vi "Disconnect Core.vi"(8 "error in (no error)":errorcluster, 10 "Force (T)":bool=TRUE, 11 "BNT_SLTagConnection in":refnum<class "BNT_SLTagConnection.lvclass">) -> (0 "error out":errorcluster, 3 "BNT_SLTagConnection out":refnum<class "BNT_SLTagConnection.lvclass">)   [LabVIEW 2019, in "BNT_SLTagConnection.lvlib" / "BNT_SLTagConnection.lvclass"]
doc: "Close reference to a process variable."
uses:
  BNT_SLTagConnection.lvclass
  BNT_SLTagConnection.lvclass/BNT_SLTagConnection.ctl
  <vilib>/Skyline/Tag/Wrapper/Wrapper_class/NI Skyline Tag.lvclass/NI Skyline Tag.ctl
  <vilib>/Skyline/Tag/Wrapper/Wrapper_class/NI Skyline Tag.lvclass
  <vilib>/Skyline/Tag/Wrapper/Wrapper_class/Read Tag Path.vi
  <vilib>/Skyline/Tag/Wrapper/Wrapper_class/Close Tag (Single).vi
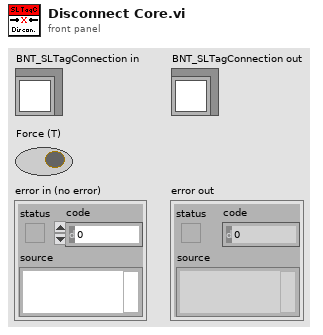
[diagram p1: front panel]
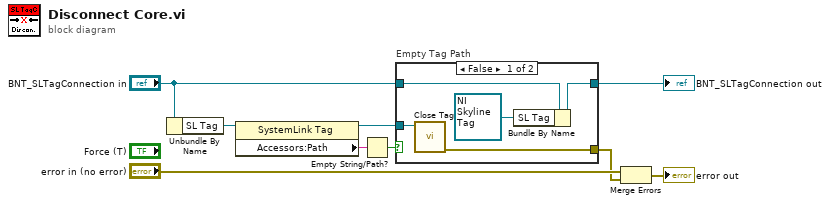
[diagram p0: block diagram]
diagram:
  n1 = Unbundle By Name("BNT_SLTagConnection in") -> ("SL Tag"=w3:refnum<class "NI Skyline Tag.lvclass">)
  n2 = property class="SystemLink Tag"(reference=w3) -> (reference out=w2:refnum<class "NI Skyline Tag.lvclass">, "Accessors:Path"=w1:string)  [unwired: 1 in, 1 out]
  n3 = Empty String/Path?(string/path=w1) -> (empty?=w7:bool)
  n4 = case "Empty Tag Path" shown="False" w7 {
    tunnel: w2 -> [w14 _]
    tunnel: [w13 _] -> w4
    tunnel: "BNT_SLTagConnection in" -> [w12 w15]
    tunnel: [w11 w15] -> w8
    frame False {
      n5 = call-poly <vilib>:"Close Tag.vi"("tag"=w14) -> ("error out"=w13:errorcluster)  [unwired: 10 in]
      n6 = Bundle By Name(cluster=w12, "SL Tag"=refnum<class "NI Skyline Tag.lvclass"> refnum ("Tag")) -> (w11:refnum<class "BNT_SLTagConnection.lvclass">)
    }
    frame True {
    }
  }
  "BNT_SLTagConnection out" <- w8
  n7 = Merge Errors("error in (no error)", w4) -> (→"error out":errorcluster)
